vi "Self Alias.vi"(11 "jettl in":refnum<class "jettl.lvclass">) -> (0 "error out":errorcluster, 2 "Alias":string)   [LabVIEW 2021, in "jettl.lvlib" / "jettl.lvclass"]
uses:
  jettl.lvclass
  jettl.lvclass/jettl.ctl
  jettl.lvlib
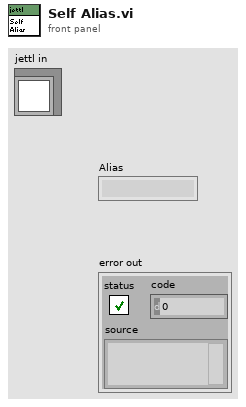
[diagram p1: front panel]
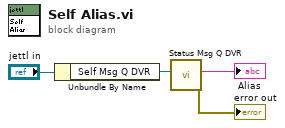
[diagram p0: block diagram]
diagram:
  n1 = Unbundle By Name("jettl in") -> ("Self Msg Q DVR"=w3:refnum<data-value>)
  n2 = call "Status Msg Q DVR.vi"("Msg Q DVR"=w3) -> ("error out"=→"error out":errorcluster, "Msg Q DVR Alias"=→"Alias":string)  [unwired: 9 in]
